vi "Logging_SubVI.vi"(9 "timestamp":timestamp, 10 "Array":dbl[](array[numeric]), 11 "file path (dialog if empty)":path) -> ()   [LabVIEW 2012]
uses:
  <vilib>/Utility/file.llb/Write To Spreadsheet File (string).vi
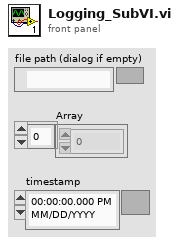
[diagram p1: front panel]
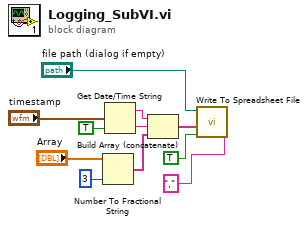
[diagram p0: block diagram]
diagram:
  n1 = Number To Fractional String(number="Array", precision (6)=i16 3) -> (F-format string=w6:string[])  [unwired: 2 in]
  n2 = Get Date/Time String(seconds (now)="timestamp", want seconds? (F)=TRUE) -> (date string=w11:string, time string=w10:string)  [unwired: 1 in]
  n3 = Build Array (concatenate)(w11, w10, w6) -> (w7:string[])
  n4 = call-poly <vilib>:"Write To Spreadsheet File.vi"("delimiter (\\t)"="," ("delimiter (\\t)"), "append to file? (new file:F)"=TRUE, "1D data"=w7, "file path (dialog if empty)"="file path (dialog if empty)") -> ()  [unwired: 4 in, 1 out]
